vi "write_notifiers_to_string.vi"(10 "Mission Notifiers":T2, 11 "NotifierReff":T1) -> (3 "input cluster":cluster{"names":string, "value":variant})   [LabVIEW 2013]
doc: "Converts all notifiers to a string"
uses:
  Data/TypeDefs/MissionNotifiers.ctl
  Logic/Classes/Missions/GenericMission/GenericMission.lvclass
  Logic/Classes/Obstacle/Obstacle.lvclass
  Data/TypeDefs/Notifiers.ctl
  Data/TypeDefs/UTM Location.ctl
  Data/TypeDefs/Sail Set Suggestions.ctl
  Data/TypeDefs/Rudder Set Suggestions.ctl
  Data/TypeDefs/OverrideInformation.ctl
  Data/TypeDefs/OverrideMode.ctl
  Data/TypeDefs/MotorSetup.ctl
  Data/TypeDefs/DynamixelSetupInfo.ctl
  Data/TypeDefs/AirmarStatus.ctl
  Data/TypeDefs/HardwareOnline.ctl
  Data/TypeDefs/DynamixelCycleTracker.ctl
  Data/TypeDefs/RC Input Values.ctl
  Logic/Classes/Waypoint/Waypoint.lvclass
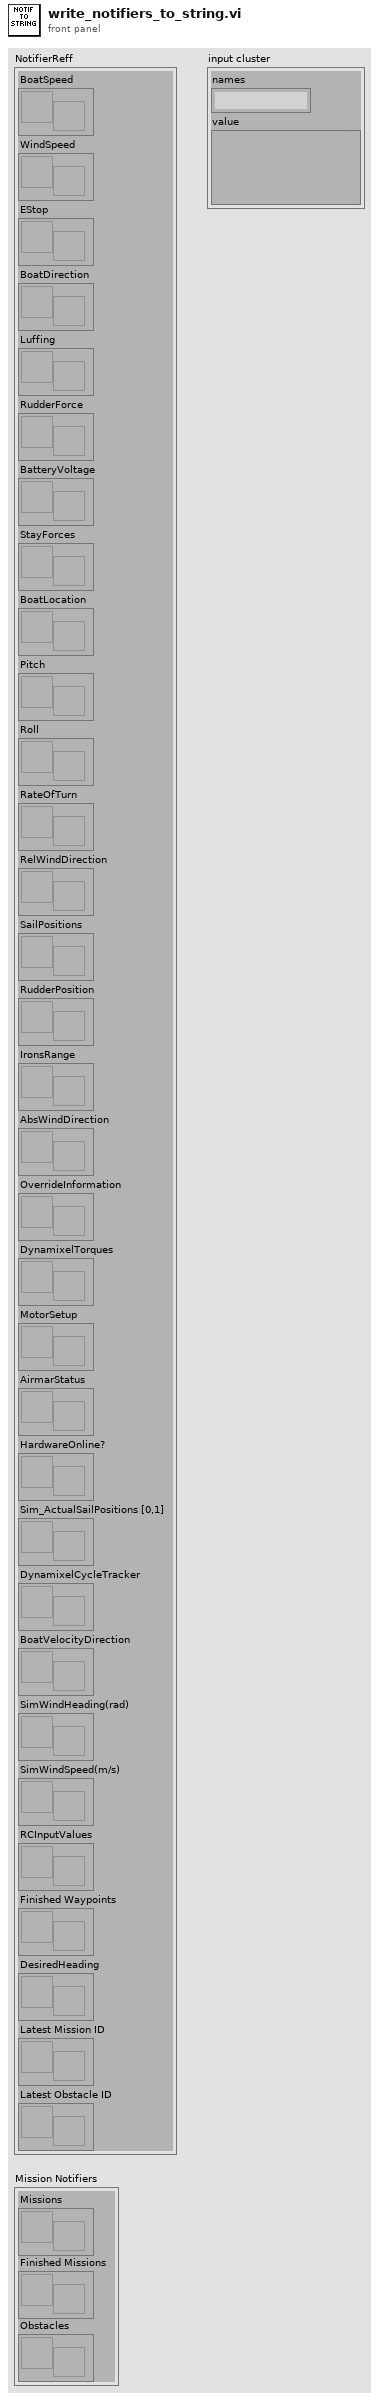
[diagram p1: front panel]
types:
  T1 = typedef "Notifiers.ctl" = cluster{"BoatSpeed":refnum<notifier>, "WindSpeed":refnum<notifier>, "EStop":refnum<notifier>, "BoatDirection":refnum<notifier>, "Luffing":refnum<notifier>, "RudderForce":refnum<notifier>, "BatteryVoltage":refnum<notifier>, "StayForces":refnum<notifier>, "BoatLocation":refnum<notifier>, "Pitch":refnum<notifier>, "Roll":refnum<notifier>, "RateOfTurn":refnum<notifier>, "RelWindDirection":refnum<notifier>, "SailPositions":refnum<notifier>, "RudderPosition":refnum<notifier>, "IronsRange":refnum<notifier>, "AbsWindDirection":refnum<notifier>, "OverrideInformation":refnum<notifier>, "DynamixelTorques":refnum<notifier>, "MotorSetup":refnum<notifier>, "AirmarStatus":refnum<notifier>, "HardwareOnline?":refnum<notifier>, "Sim_ActualSailPositions [0,1]":refnum<notifier>, "DynamixelCycleTracker":refnum<notifier>, "BoatVelocityDirection":refnum<notifier>, "SimWindHeading(rad)":refnum<notifier>, "SimWindSpeed(m/s)":refnum<notifier>, "RCInputValues":refnum<notifier>, "Finished Waypoints":refnum<notifier>, "DesiredHeading":refnum<notifier>, "Latest Mission ID":refnum<notifier>, "Latest Obstacle ID":refnum<notifier>}
  T2 = typedef "MissionNotifiers.ctl" = cluster{"Missions":refnum<notifier>, "Finished Missions":refnum<notifier>, "Obstacles":refnum<notifier>}
  T3 = typedef "HardwareOnline.ctl" = cluster{"AirmarOnline":bool, "WindvaneOnline":bool, "HemisphereOnline":bool, "StayForceOnline":bool, "BatteryVoltageOnline":bool, "AccelerometerOnline":bool, "MainDynamixel Online":bool, "JibDynamixel Online":bool, "RudderDynamixel Online":bool}
  T4 = typedef "MotorSetup.ctl" = cluster{"Main Dynamixel Set Data":T5, "Rudder Dynamixel Set Data":T5, "Jib Dynamixel Set Data":T5}
  T5 = typedef "DynamixelSetupInfo.ctl" = cluster{"Lower Winch Bound (deg)":dbl, "Upper Winch Bound (deg)":dbl}
  T6 = typedef "OverrideInformation.ctl" = cluster{"OverrideMode":T7, "SailSetting":T8, "Rudder Setpoint":T9, "Sim_Wind_Speed":dbl, "Sim_Wind_Heading":dbl}
  T7 = typedef "OverrideMode.ctl" = enum16{"None", "Rudder", "Sails", "Both"}
  T8 = typedef "Sail Set Suggestions.ctl" = cluster{"MainSailSuggestion":dbl, "JibSailSuggestion":dbl}
  T9 = typedef "Rudder Set Suggestions.ctl" = dbl
  T10 = typedef "UTM Location.ctl" = cluster{"UTM Zone":dbl, "Hemisphere":enum16{"North", "South"}, "East":dbl, "North":dbl}
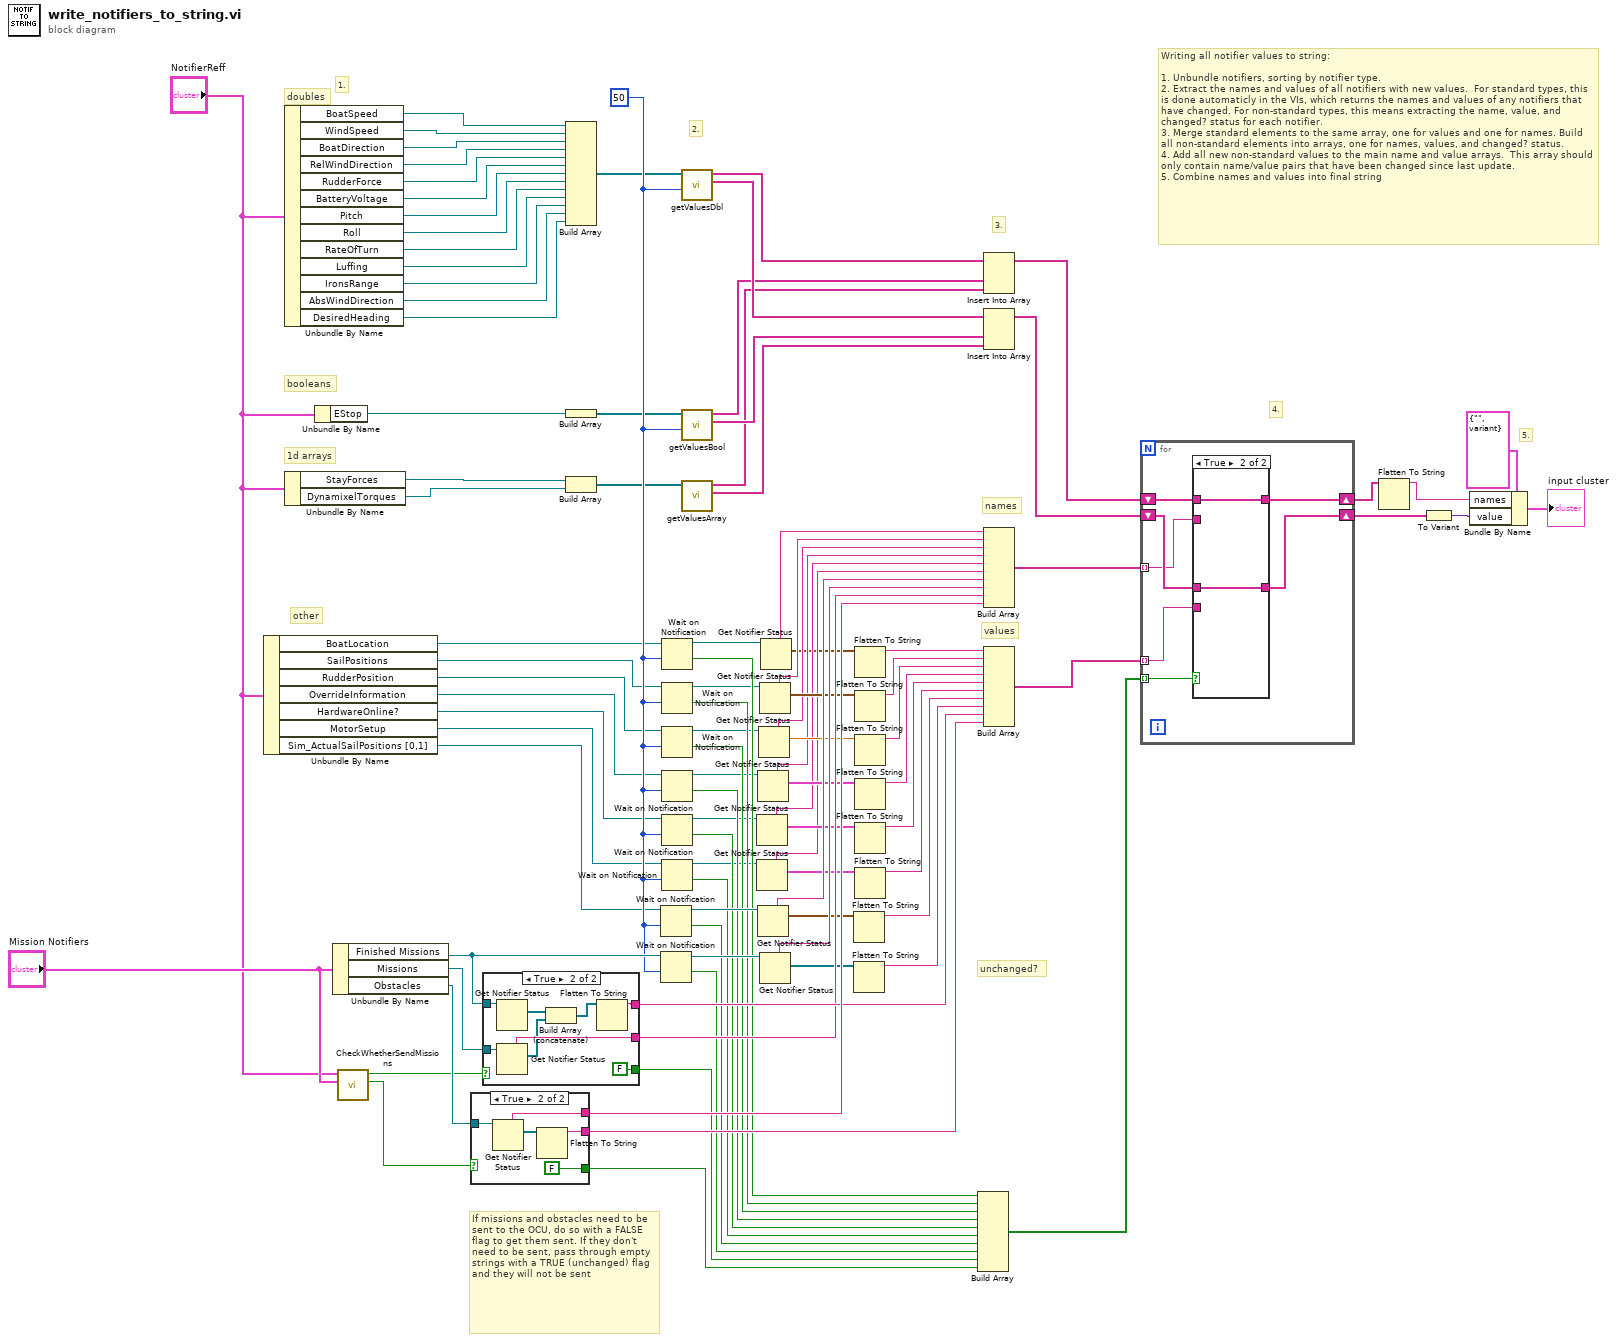
[diagram p0: block diagram]
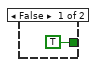
[diagram p2: hidden frame]
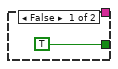
[diagram p3: hidden frame]
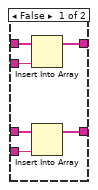
[diagram p4: hidden frame]
diagram:
  w83 = 50 ("timeout in ms (-1)")
  # "5."
  # "If missions and obstacles need to be sent to the OCU, do so with a FALSE flag to get them sent. If they don't need to be sent, pass through empty strings with a TRUE (unchanged) flag and they will not be sent"
  # "Writing all notifier values to string:\n\n1. Unbundle notifiers, sorting by notifier type.\n2. Extract the names and values of all notifiers with new values.  For standard types, this is done automaticly in the VIs, which returns the names and values of any notifiers that have changed. For non-standard types, this means extracting the name, value, and changed? status for each notifier. \n3. Merge standard elements to the same array, one for values and one for names. Build all non-standard elements into arrays, one for names, values, and changed? status.\n4. Add all new non-standard values to the main name and value arrays.  This array should only contain name/value pairs that have been changed since last update.\n5. Combine names and values into final string"
  # "4."
  # "3."
  # "2."
  # "1."
  # "unchanged?"
  # "values"
  # "names"
  # "other"
  # "1d arrays"
  # "booleans"
  # "doubles"
  n1 = Unbundle By Name("NotifierReff") -> ("BoatLocation"=w13:refnum<notifier>, "SailPositions"=w14:refnum<notifier>, "RudderPosition"=w15:refnum<notifier>, "OverrideInformation"=w17:refnum<notifier>, "HardwareOnline?"=w16:refnum<notifier>, "MotorSetup"=w18:refnum<notifier>, "Sim_ActualSailPositions [0,1]"=w69:refnum<notifier>)
  n2 = Unbundle By Name("NotifierReff") -> ("BoatSpeed"=w82:refnum<notifier>, "WindSpeed"=w81:refnum<notifier>, "BoatDirection"=w1:refnum<notifier>, "RelWindDirection"=w84:refnum<notifier>, "RudderForce"=w2:refnum<notifier>, "BatteryVoltage"=w3:refnum<notifier>, "Pitch"=w4:refnum<notifier>, "Roll"=w5:refnum<notifier>, "RateOfTurn"=w6:refnum<notifier>, "Luffing"=w7:refnum<notifier>, "IronsRange"=w8:refnum<notifier>, "AbsWindDirection"=w9:refnum<notifier>, "DesiredHeading"=w80:refnum<notifier>)
  n3 = Unbundle By Name("NotifierReff") -> ("StayForces"=w12:refnum<notifier>, "DynamixelTorques"=w11:refnum<notifier>)
  n4 = Unbundle By Name("NotifierReff") -> ("EStop"=w10:refnum<notifier>)
  n5 = Unbundle By Name("Mission Notifiers") -> ("Finished Missions"=w97:refnum<notifier>, "Missions"=w87:refnum<notifier>, "Obstacles"=w92:refnum<notifier>)
  n6 = call "CheckWhetherSendMissions.vi"("Mission Notifiers"="Mission Notifiers", "NotifierReff"="NotifierReff") -> ("Send obstacles?"=w93:bool, "Send missions?"=w88:bool)  [unwired: 8 in]
  n7 = case shown="True" w93 {
    tunnel: w92 -> [_ w103]
    tunnel: [_ w102] -> w94
    tunnel: [_ w100] -> w95
    tunnel: [TRUE FALSE] -> w96
    frame False {
    }
    frame True {
      n8 = Get Notifier Status(notifier=w103) -> (notifier name=w102:string, current notification=w101:refnum<class "Obstacle.lvclass">[])  [unwired: 1 in, 3 out]
      n9 = Flatten To String(anything=w101) -> (data string=w100:string)  [unwired: 3 in, 2 out]
    }
  }
  n10 = case shown="True" w88 {
    tunnel: w87 -> [_ w110]
    tunnel: [_ w108] -> w89
    tunnel: [_ w112] -> w90
    tunnel: [TRUE FALSE] -> w91
    tunnel: w97 -> [_ w109]
    frame False {
    }
    frame True {
      n11 = Get Notifier Status(notifier=w109) -> (current notification=w107:refnum<class "GenericMission.lvclass">[])  [unwired: 1 in, 4 out]
      n12 = Get Notifier Status(notifier=w110) -> (notifier name=w108:string, current notification=w105:refnum<class "GenericMission.lvclass">[])  [unwired: 1 in, 3 out]
      n13 = Build Array (concatenate)(w107, w105) -> (w106:refnum<class "GenericMission.lvclass">[])
      n14 = Flatten To String(anything=w106) -> (data string=w112:string)  [unwired: 3 in, 2 out]
    }
  }
  n15 = Build Array(w82, w81, w1, w84, w2, w3, w4, w5, w6, w7, w8, w9, w80) -> (w25:refnum<notifier>[])
  n16 = Build Array(w10) -> (w26:refnum<notifier>[])
  n17 = Build Array(w12, w11) -> (w27:refnum<notifier>[])
  n18 = Wait on Notification(notifier=w69, timeout in ms (-1)=w83) -> (notifier out=w70:refnum<notifier>, timed out?=w74:bool)  [unwired: 2 in, 2 out]
  n19 = Wait on Notification(notifier=w97, timeout in ms (-1)=w83) -> (notifier out=w76:refnum<notifier>, timed out?=w75:bool)  [unwired: 2 in, 2 out]
  n20 = Wait on Notification(notifier=w13, timeout in ms (-1)=w83) -> (notifier out=w28:refnum<notifier>, timed out?=w51:bool)  [unwired: 2 in, 2 out]
  n21 = Wait on Notification(notifier=w14, timeout in ms (-1)=w83) -> (notifier out=w31:refnum<notifier>, timed out?=w50:bool)  [unwired: 2 in, 2 out]
  n22 = Wait on Notification(notifier=w15, timeout in ms (-1)=w83) -> (notifier out=w33:refnum<notifier>, timed out?=w49:bool)  [unwired: 2 in, 2 out]
  n23 = Wait on Notification(notifier=w17, timeout in ms (-1)=w83) -> (notifier out=w35:refnum<notifier>, timed out?=w48:bool)  [unwired: 2 in, 2 out]
  n24 = Wait on Notification(notifier=w16, timeout in ms (-1)=w83) -> (notifier out=w37:refnum<notifier>, timed out?=w47:bool)  [unwired: 2 in, 2 out]
  n25 = Wait on Notification(notifier=w18, timeout in ms (-1)=w83) -> (notifier out=w39:refnum<notifier>, timed out?=w46:bool)  [unwired: 2 in, 2 out]
  n26 = call "getValuesDbl.vi"("timeout in ms (-1)"=w83, "notifiers in"=w25) -> ("notifier values"=w55:string[], "notifier names"=w52:string[])  [unwired: 7 in, 1 out]
  n27 = call "getValuesBool.vi"("timeout in ms (-1)"=w83, "notifiers in"=w26) -> ("notifier values"=w56:string[], "notifier names"=w53:string[])  [unwired: 7 in, 1 out]
  n28 = call "getValuesArray.vi"("appended array"=w27) -> ("notifier values"=w57:string[], "notifier names"=w54:string[])  [unwired: 8 in, 1 out]
  n29 = Get Notifier Status(notifier=w37) -> (notifier name=w38:string, current notification=w44:T3)  [unwired: 1 in, 3 out]
  n30 = Get Notifier Status(notifier=w39) -> (notifier name=w40:string, current notification=w45:T4)  [unwired: 1 in, 3 out]
  n31 = Get Notifier Status(notifier=w35) -> (notifier name=w36:string, current notification=w43:T6)  [unwired: 1 in, 3 out]
  n32 = Get Notifier Status(notifier=w70) -> (notifier name=w73:string, current notification=w71:T8)  [unwired: 1 in, 3 out]
  n33 = Get Notifier Status(notifier=w33) -> (notifier name=w34:string, current notification=w42:T9)  [unwired: 1 in, 3 out]
  n34 = Get Notifier Status(notifier=w31) -> (notifier name=w32:string, current notification=w41:T8)  [unwired: 1 in, 3 out]
  n35 = Get Notifier Status(notifier=w76) -> (notifier name=w77:string, current notification=w78:refnum<class "GenericMission.lvclass">[])  [unwired: 1 in, 3 out]
  n36 = Get Notifier Status(notifier=w28) -> (notifier name=w30:string, current notification=w29:T10)  [unwired: 1 in, 3 out]
  n37 = Flatten To String(anything=w71) -> (data string=w72:string)  [unwired: 3 in, 2 out]
  n38 = Flatten To String(anything=w78) -> (data string=w79:string)  [unwired: 3 in, 2 out]
  n39 = Flatten To String(anything=w29) -> (data string=w19:string)  [unwired: 3 in, 2 out]
  n40 = Flatten To String(anything=w41) -> (data string=w20:string)  [unwired: 3 in, 2 out]
  n41 = Flatten To String(anything=w42) -> (data string=w21:string)  [unwired: 3 in, 2 out]
  n42 = Flatten To String(anything=w43) -> (data string=w22:string)  [unwired: 3 in, 2 out]
  n43 = Flatten To String(anything=w44) -> (data string=w23:string)  [unwired: 3 in, 2 out]
  n44 = Flatten To String(anything=w45) -> (data string=w24:string)  [unwired: 3 in, 2 out]
  n45 = Build Array(w51, w50, w49, w48, w47, w46, w74, w75, w91, w96) -> (w60:bool[])
  n46 = Insert Into Array(array=w52, new element #1=w53, new element #2=w54) -> (w58:string[])  [unwired: 1 in]
  n47 = Insert Into Array(array=w55, new element #1=w56, new element #2=w57) -> (w59:string[])  [unwired: 1 in]
  n48 = Build Array(w30, w32, w34, w36, w38, w40, w73, w77, w89, w94) -> (w61:string[])
  n49 = Build Array(w19, w20, w21, w22, w23, w24, w72, w79, w90, w95) -> (w62:string[])
  n50 = for {
    tunnel: w60 -> [w119] mode=indexing
    shift-right: [w118] -> w67
    shift-left: w58 -> [w113]
    shift-right: [w116] -> w63
    shift-left: w59 -> [w117]
    tunnel: w61 -> [w115] mode=indexing
    tunnel: w62 -> [w114] mode=indexing
    n51 = case shown="True" w119 {
      tunnel: [w125 w126] -> w118
      tunnel: w117 -> [w124 w127]
      tunnel: [w123 w127] -> w116
      tunnel: w115 -> [w122 _]
      tunnel: w114 -> [w121 _]
      tunnel: w113 -> [w120 w126]
      frame False {
        n52 = Insert Into Array(array=w120, new element=w122) -> (w125:string[])  [unwired: 1 in]
        n53 = Insert Into Array(array=w124, new element=w121) -> (w123:string[])  [unwired: 1 in]
      }
      frame True {
      }
    }
  }
  n54 = Flatten To String(anything=w67) -> (data string=w68:string)  [unwired: 3 in, 2 out]
  n55 = To Variant(anything=w63) -> (Variant=w66:variant)
  n56 = Bundle By Name(cluster=cluster{"names":string, "value":variant} {"names"="", "value"=variant} ("input cluster"), "names"=w68, "value"=w66) -> (→"input cluster":cluster{"names":string, "value":variant})
